vi "get globally unique identifier.vi"(8 "error in (no error)":errorcluster, 10 "globally_unique_identifier":T1, 11 "id":i32) -> (0 "error out":errorcluster, 2 "globally_unique_identifier out":T1, 3 "function return":i32)   [LabVIEW 2012, in "libximc.lvlib"]
doc: "result_t XIMC_API get_globally_unique_identifier (device_t id, globally_unique_identifier_t* globally_unique_identifier);"
uses:
  libximc.lvlib
  libximc.dll
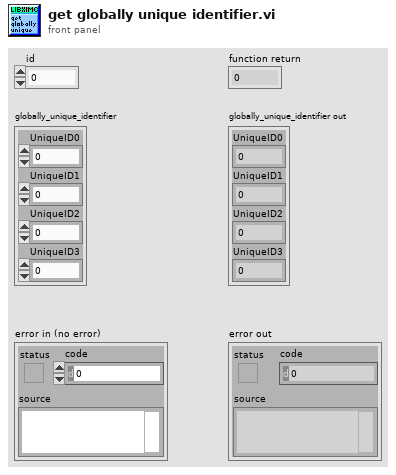
[diagram p1: front panel]
types:
  T1 = cluster{"UniqueID0":u32, "UniqueID1":u32, "UniqueID2":u32, "UniqueID3":u32}
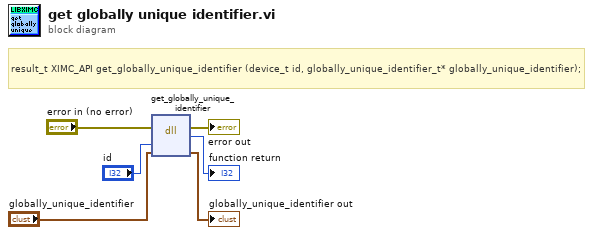
[diagram p0: block diagram]
diagram:
  # "result_t XIMC_API get_globally_unique_identifier (device_t id, globally_unique_identifier_t* globally_unique_identifier);"
  n1 = dll-call lib="E:/labview-2.12.1-Labview_12.0/ximcLVx32/libximc.*" fn="get_globally_unique_identifier"(error in="error in (no error)", "id"="id", "globally_unique_identifier"="globally_unique_identifier") -> (error out=→"error out":errorcluster, →"function return":i32, "globally_unique_identifier"=→"globally_unique_identifier out":T1)  [unwired: 3 in, 1 out]
